vi "Check for Reboot Loop.vi"(8 "error in (no error)":errorcluster caption="错误输入（无错误）") -> (0 "error out":errorcluster caption="错误输出", 2 "Start in Safe Mode?":bool caption="在安全模式中启动？")   [LabVIEW 2013]
uses:
  Globals/Global - Configuration Options.vi
  <vilib>/Utility/file.llb/Read From Spreadsheet File (string).vi
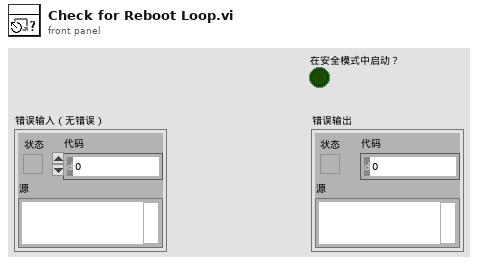
[diagram p1: front panel]
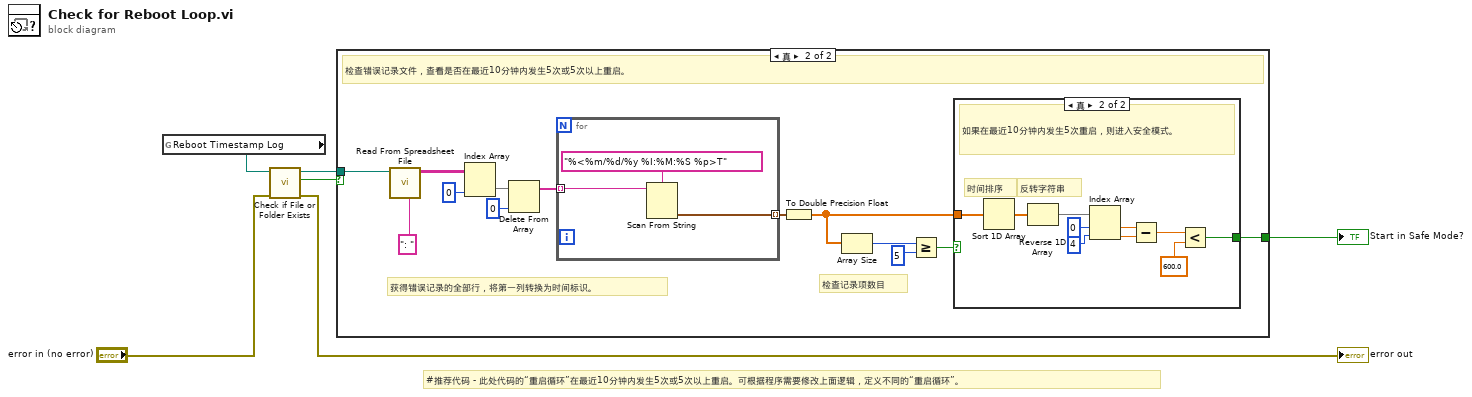
[diagram p0: block diagram]
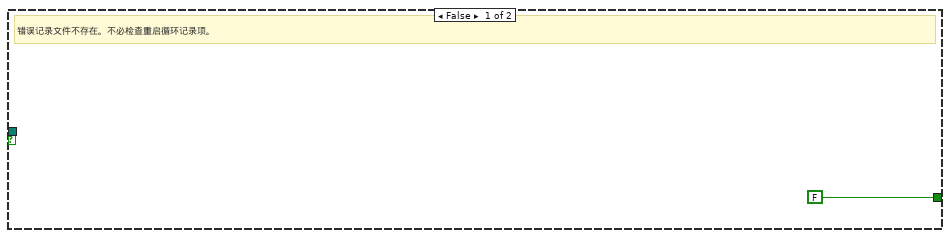
[diagram p2: hidden frame]
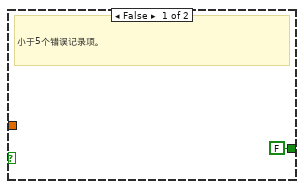
[diagram p3: hidden frame]
diagram:
  # "#推荐代码 - 此处代码的“重启循环”在最近10分钟内发生5次或5次以上重启。可根据程序需要修改上面逻辑，定义不同的“重启循环”。"
  n1 = global read "Global - Configuration Options.vi" "Reboot Timestamp Log"() -> (w1:path)
  n2 = call <vilib>:"Check if File or Folder Exists.vi"("error in (no error)"="error in (no error)", "path"=w1) -> ("error out"=→"error out":errorcluster, "file or folder exists?"=w4:bool, "dup path"=w3:path)  [unwired: 7 in]
  n3 = case shown="真" w4 {
    tunnel: w3 -> [_ w20]
    tunnel: [FALSE w16] -> w2
    frame False {
      # "错误记录文件不存在。不必检查重启循环记录项。"
    }
    frame True {
      # "检查记录项数目"
      # "获得错误记录的全部行，将第一列转换为时间标识。"
      # "检查错误记录文件，查看是否在最近10分钟内发生5次或5次以上重启。"
      n4 = call-poly <vilib>:"Read From Spreadsheet File.vi"("delimiter (\\t)"=": " ("delimiter (\\t)"), "file path (dialog if empty)"=w20) -> ("all rows"=w19:string[][])  [unwired: 5 in, 4 out]
      n5 = Index Array(array=w19, index (col)=0 ("disabled index (col)")) -> (element=w10:string[])  [unwired: 1 in]
      n6 = Delete From Array(array=w10, index=0) -> (array with subset deleted=w9:string[])  [unwired: 1 in, 1 out]
      n7 = for {
        tunnel: w9 -> [w34] mode=indexing
        tunnel: [w33] -> w17 mode=indexing
        n8 = Scan From String(format string="%<%m/%d/%y %I:%M:%S %p>T", input string=w34) -> (output 1=w33:timestamp)  [unwired: 3 in, 3 out]
      }
      n9 = To Double Precision Float(number=w17) -> (double precision float=w15:dbl[])
      n10 = Array Size(array=w15) -> (size(s)=w14:i32)
      n11 = Greater Or Equal?(x=w14, y=5) -> (x >= y?=w12:bool)
      n12 = case shown="真" w12 {
        tunnel: [FALSE w23] -> w16
        tunnel: w15 -> [_ w22]
        frame False {
          # "小于5个错误记录项。"
        }
        frame True {
          # "反转字符串"
          # "时间排序"
          # "如果在最近10分钟内发生5次重启，则进入安全模式。"
          n13 = Sort 1D Array(array=w22) -> (sorted array=w31:dbl[])
          n14 = Reverse 1D Array(array=w31) -> (reversed array=w30:dbl[])
          n15 = Index Array(array=w30, index #1=0 ("index"), index #2=4 ("index")) -> (element #1=w27:dbl, element #2=w26:dbl)
          n16 = Subtract(x=w27, y=w26) -> (x-y=w25:dbl)
          n17 = Less?(x=w25, y=600.0) -> (x < y?=w23:bool)
        }
      }
    }
  }
  "Start in Safe Mode?" <- w2
